vi "Self.vi"(9 "Is Priority":bool, 10 "Msg":refnum<class "Msg.lvclass">, 11 "Base Actor in":refnum<class "Base Actor.lvclass">) -> (3 "Base Actor out":refnum<class "Base Actor.lvclass">)   [LabVIEW 2021, in "jettl.lvlib" / "Actor.lvlib" / "Base Actor.lvclass"]
uses:
  Base Actor.lvclass
  Msg/Msg.lvclass
  Sender/Relation.ctl
  Base Actor.lvclass/Base Actor.ctl
  Sender/Sender.lvlib
  Error/Error.lvlib
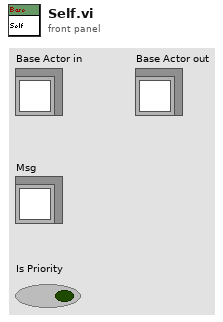
[diagram p1: front panel]
types:
  T1 = typedef "jettl.lvlib/Actor.lvlib/Implemented Msgs.ctl" = set{refnum<class "Msg.lvclass">}
  T2 = typedef "jettl.lvlib/Sender.lvlib/Relation.ctl" = enum16{"Self", "Creator", "Created"}
  T3 = typedef "jettl.lvlib/Actor.lvlib/Attributes.ctl" = cluster{"Alias":string, "Address":refnum<user-event>, "Implemented Msgs":T1, "Path":path}
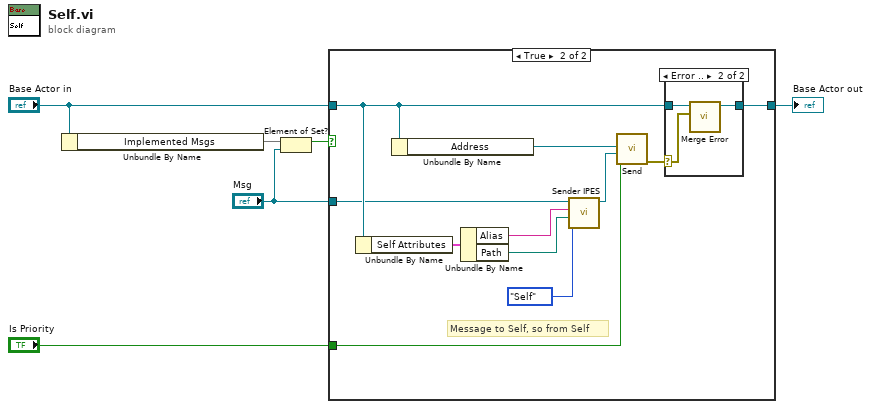
[diagram p0: block diagram]
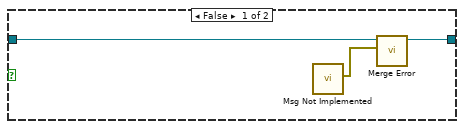
[diagram p2: hidden frame]
diagram:
  n1 = Unbundle By Name("Base Actor in") -> ("Implemented Msgs"=w3:T1)
  n2 = Element of Set?(10:"Msg", 11:w3) -> (3:w1:bool)
  n3 = case shown="True" w1 {
    tunnel: [w8 w20] -> w6
    tunnel: "Is Priority" -> [_ w19]
    tunnel: "Base Actor in" -> [w9 w11]
    tunnel: "Msg" -> [_ w10]
    frame False {
      n4 = call "Msg Not Implemented.vi"() -> ("Error"=w7:errorcluster)  [unwired: 11 in]
      n5 = call-dynamic "Merge Error.vi"("Error"=w7, "Base Actor in"=w9) -> ("Base Actor out"=w8:refnum<class "Base Actor.lvclass">)  [unwired: 9 in]
    }
    frame True {
      # "Message to Self, so from Self"
      n6 = Unbundle By Name(w11) -> ("Self Attributes"=w16:T3)
      n7 = Unbundle By Name(w11) -> ("Address"=w17:refnum<user-event>)
      n8 = Unbundle By Name(w16) -> ("Alias"=w14:string, "Path"=w13:path)
      n9 = call "Sender IPES.vi"("Relation"=Relation."Self", "Path"=w13, "Self Alias"=w14, "Msg in"=w10) -> ("Msg out"=w15:refnum<class "Msg.lvclass">)  [unwired: 7 in]
      n10 = call "Send.vi"("Is Priority"=w19, "Msg"=w15, "Address"=w17) -> ("error out"=w18:errorcluster)  [unwired: 8 in]
      n11 = case shown="Error .." w18 {
        selector: w18 -> [_ w22]
        tunnel: [w21 w24] -> w20
        tunnel: w11 -> [w21 w23]
        frame No Error {
        }
        frame Error {
          n12 = call-dynamic "Merge Error.vi"("Error"=w22, "Base Actor in"=w23) -> ("Base Actor out"=w24:refnum<class "Base Actor.lvclass">)  [unwired: 9 in]
        }
      }
    }
  }
  "Base Actor out" <- w6
